vi "onUnhandledDependencyError.vi"(7 "(deprecated -- use Handle Error override)":bool, 8 "Unhandled Dependency Error":errorcluster, 9 "Dependency":refnum<class "SMO.lvclass">, 11 "SMO in":refnum<class "SMO.lvclass">) -> (0 "Unhandled error":errorcluster, 3 "SMO out":refnum<class "SMO.lvclass">)   [LabVIEW 2021, in "smo.lvlib" / "SMO.lvclass"]
uses:
  SMO.lvclass
  SMO.lvclass/SMO.ctl
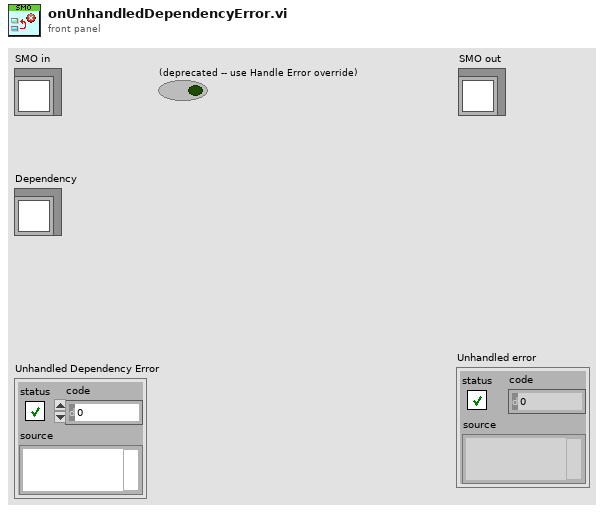
[diagram p1: front panel]
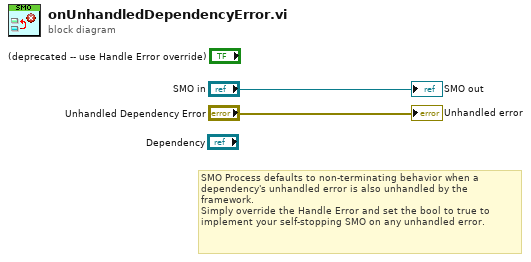
[diagram p0: block diagram]
diagram:
  # "SMO Process defaults to non-terminating behavior when a dependency's unhandled error is also unhandled by the framework.\nSimply override the Handle Error and set the bool to true to implement your self-stopping SMO on any unhandled error."
  "SMO out" <- "SMO in"
  "Unhandled error" <- "Unhandled Dependency Error"
